vi "OneForAll.vi"() -> ()   [LabVIEW 2019]
uses:
  <vilib>/Rock Robotics/WPI/ThirdParty/Phoenix-LabVIEW/Motor Controller/Controls/CTRE_Phoenix_MotorControl_ControlMode.ctl
panel:
  in  "malgeza":dbl
  in  "Intake":dbl
  in  "elevator":dbl
  in  "shooter":dbl
  in  "loader":dbl
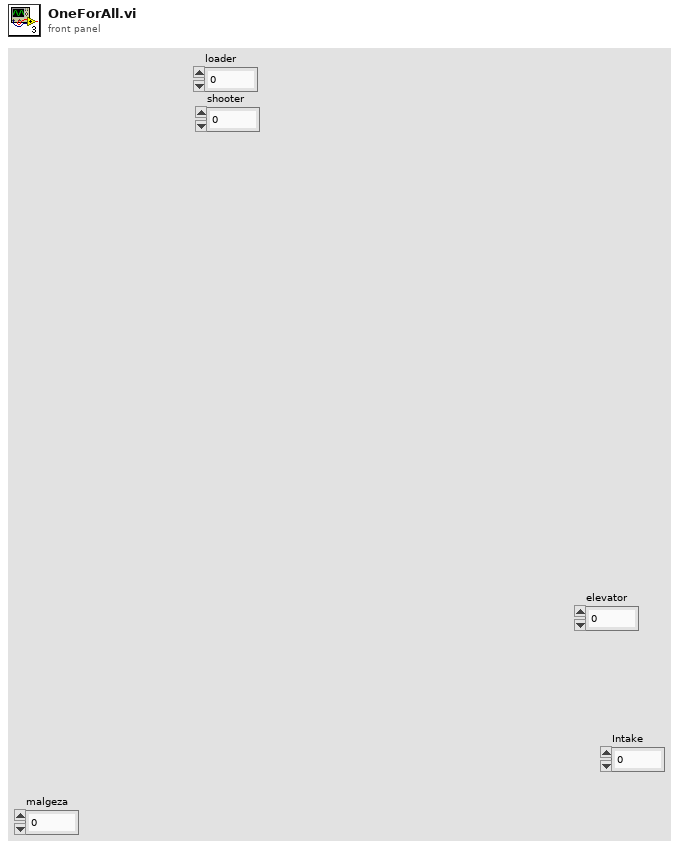
[diagram p1: front panel]
types:
  T1 = typedef "WPI_MotorControlDeviceRef.ctl" = cluster{"DeviceStatus":errorcluster, "Type":T2, "PWM":cluster{"PWM Channel":T3, "DeadBand":T4}, "CAN":cluster{"Device Number":u8, "SetOutput VI Ref":variant, "GetOutput VI Ref":variant, "Enable VI Ref":variant, "Disable VI Ref":variant, "Data":variant}, "Invert":bool, "DIO PWM":cluster{"PWM \"Enable\" Channel":T3, "DIOChannel":T5, "PWM Rate":dbl}}
  T2 = typedef "WPI_MotorControlType.ctl" = enum16{"PWM", "CAN", "DIO PWM"}
  T3 = typedef "FPGA_DIOPWMChannel.ctl" = enum8{"PWM 0", "PWM 1", "PWM 2", "PWM 3", "PWM 4", "PWM 5", "PWM 6", "PWM 7", "PWM 8", "PWM 9", "PWM MXP 0", "PWM MXP 1", "PWM MXP 2", "PWM MXP 3", "PWM MXP 4", "PWM MXP 5", "PWM MXP 6", "PWM MXP 7", "PWM MXP 8", "PWM MXP 9", "Invalid"}
  T4 = typedef "WPI_PWMDeadband.ctl" = cluster{"Name":string, "maxPositivePwm":i32, "minPositivePwm":i32, "centerPwm":i32, "maxNegativePwm":i32, "minNegativePwm":i32, "angularRange":u16}
  T5 = typedef "FPGA_DIOChannel.ctl" = enum8{"DIO 0", "DIO 1", "DIO 2", "DIO 3", "DIO 4", "DIO 5", "DIO 6", "DIO 7", "DIO 8", "DIO 9", "DIO MXP 0", "DIO MXP 1", "DIO MXP 2", "DIO MXP 3", "DIO MXP 4", "DIO MXP 5", "DIO MXP 6", "DIO MXP 7", "DIO MXP 8", "DIO MXP 9", "DIO MXP 10", "DIO MXP 11", "DIO MXP 12", "DIO MXP 13", "DIO MXP 14", "DIO MXP 15", "SPI Port CS1", "SPI Port CS2", "SPI Port CS3", "SPI Port MISO", "SPI Port MOSI", "Invalid"}
  T6 = typedef "CTRE_Phoenix_MotorControl_ControlMode.ctl" = u16
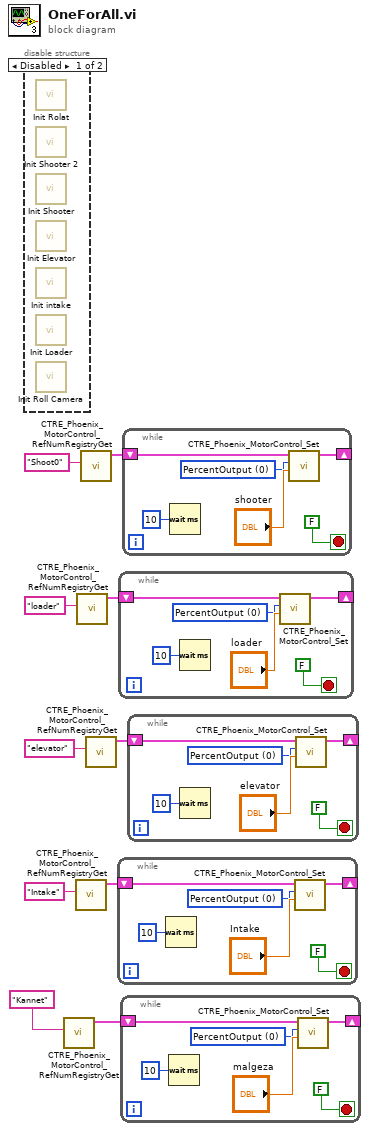
[diagram p0: block diagram]
diagram:
  n1 = disable-structure shown="Disabled" {
    frame Disabled {
      n2 = call "Init Rolat.vi"() -> ()  [unwired: 12 in]
      n3 = call "Init Shooter 2.vi"() -> ()  [unwired: 12 in]
      n4 = call "Init Shooter.vi"() -> ()  [unwired: 12 in]
      n5 = call "Init Elevator.vi"() -> ()  [unwired: 12 in]
      n6 = call "Init intake.vi"() -> ()  [unwired: 12 in]
      n7 = call "Init Loader.vi"() -> ()  [unwired: 12 in]
      n8 = call "Init Roll Camera.vi"() -> ()  [unwired: 12 in]
    }
    frame Enabled {
    }
  }
  n9 = call <vilib>:"CTRE_Phoenix_MotorControl_RefNumRegistryGet.vi"("refnum name"="Kannet") -> ("PhoenixMotorControlDevRef"=w1:T1)  [unwired: 9 in, 1 out]
  n10 = call <vilib>:"CTRE_Phoenix_MotorControl_RefNumRegistryGet.vi"("refnum name"="Intake") -> ("PhoenixMotorControlDevRef"=w3:T1)  [unwired: 9 in, 1 out]
  n11 = call <vilib>:"CTRE_Phoenix_MotorControl_RefNumRegistryGet.vi"("refnum name"="loader") -> ("PhoenixMotorControlDevRef"=w7:T1)  [unwired: 9 in, 1 out]
  n12 = call <vilib>:"CTRE_Phoenix_MotorControl_RefNumRegistryGet.vi"("refnum name"="Shoot0") -> ("PhoenixMotorControlDevRef"=w9:T1)  [unwired: 9 in, 1 out]
  n13 = call <vilib>:"CTRE_Phoenix_MotorControl_RefNumRegistryGet.vi"("refnum name"="elevator") -> ("PhoenixMotorControlDevRef"=w5:T1)  [unwired: 9 in, 1 out]
  n14 = while {
    shift-right: [w14] -> _
    shift-left: w3 -> [w15]
    stop <- FALSE stop-if-true
    w12 = T6 0 items=["PercentOutput"=0, "Position"=1, "Velocity"=2, "Current"=3, "Follower"=5, "MotionProfile"=6, "MotionMagic"=7, "MotionProfileArc"=10, "Disabled"=15] ("Control Mode")
    n15 = Wait (ms)(milliseconds to wait=u32 10) -> ()  [unwired: 1 out]
    n16 = call <vilib>:"CTRE_Phoenix_MotorControl_Set.vi"("Output"="Intake", "Control Mode"=w12, "PhoenixMotorControlDevRef"=w15) -> ("PhoenixMotorControlDevRef"=w14:T1)  [unwired: 7 in, 1 out]
  }
  n17 = while {
    shift-right: [w20] -> _
    shift-left: w7 -> [w21]
    stop <- FALSE stop-if-true
    w18 = T6 0 items=["PercentOutput"=0, "Position"=1, "Velocity"=2, "Current"=3, "Follower"=5, "MotionProfile"=6, "MotionMagic"=7, "MotionProfileArc"=10, "Disabled"=15] ("Control Mode")
    n18 = Wait (ms)(milliseconds to wait=u32 10) -> ()  [unwired: 1 out]
    n19 = call <vilib>:"CTRE_Phoenix_MotorControl_Set.vi"("Output"="loader", "Control Mode"=w18, "PhoenixMotorControlDevRef"=w21) -> ("PhoenixMotorControlDevRef"=w20:T1)  [unwired: 7 in, 1 out]
  }
  n20 = while {
    shift-right: [w26] -> _
    shift-left: w1 -> [w27]
    stop <- FALSE stop-if-true
    w24 = T6 0 items=["PercentOutput"=0, "Position"=1, "Velocity"=2, "Current"=3, "Follower"=5, "MotionProfile"=6, "MotionMagic"=7, "MotionProfileArc"=10, "Disabled"=15] ("Control Mode")
    n21 = Wait (ms)(milliseconds to wait=u32 10) -> ()  [unwired: 1 out]
    n22 = call <vilib>:"CTRE_Phoenix_MotorControl_Set.vi"("Output"="malgeza", "Control Mode"=w24, "PhoenixMotorControlDevRef"=w27) -> ("PhoenixMotorControlDevRef"=w26:T1)  [unwired: 7 in, 1 out]
  }
  n23 = while {
    shift-right: [w32] -> _
    shift-left: w9 -> [w33]
    stop <- FALSE stop-if-true
    w30 = T6 0 items=["PercentOutput"=0, "Position"=1, "Velocity"=2, "Current"=3, "Follower"=5, "MotionProfile"=6, "MotionMagic"=7, "MotionProfileArc"=10, "Disabled"=15] ("Control Mode")
    n24 = Wait (ms)(milliseconds to wait=u32 10) -> ()  [unwired: 1 out]
    n25 = call <vilib>:"CTRE_Phoenix_MotorControl_Set.vi"("Output"="shooter", "Control Mode"=w30, "PhoenixMotorControlDevRef"=w33) -> ("PhoenixMotorControlDevRef"=w32:T1)  [unwired: 7 in, 1 out]
  }
  n26 = while {
    shift-right: [w38] -> _
    shift-left: w5 -> [w39]
    stop <- FALSE stop-if-true
    w36 = T6 0 items=["PercentOutput"=0, "Position"=1, "Velocity"=2, "Current"=3, "Follower"=5, "MotionProfile"=6, "MotionMagic"=7, "MotionProfileArc"=10, "Disabled"=15] ("Control Mode")
    n27 = Wait (ms)(milliseconds to wait=u32 10) -> ()  [unwired: 1 out]
    n28 = call <vilib>:"CTRE_Phoenix_MotorControl_Set.vi"("Output"="elevator", "Control Mode"=w36, "PhoenixMotorControlDevRef"=w39) -> ("PhoenixMotorControlDevRef"=w38:T1)  [unwired: 7 in, 1 out]
  }
